vi "add data to plot 1.vi"(8 "error in (no error)":errorcluster, 9 "Input graph":cluster{"Y":dbl[], "Y":dbl[]}[](array[cluster]), 10 "Input Y array":dbl[](array[numeric]), 11 "x":dbl) -> (0 "error in (no error) 2":errorcluster, 3 "Output graph":cluster{dbl[], dbl[]}[](array[cluster]))   [LabVIEW 2024]
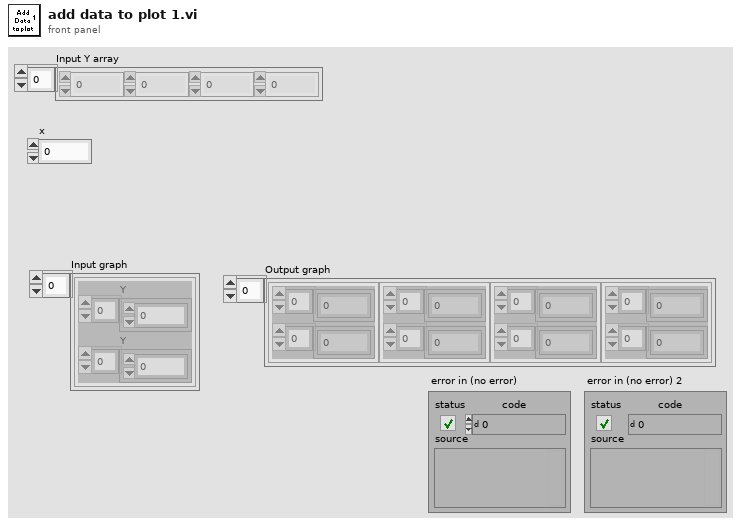
[diagram p1: front panel]
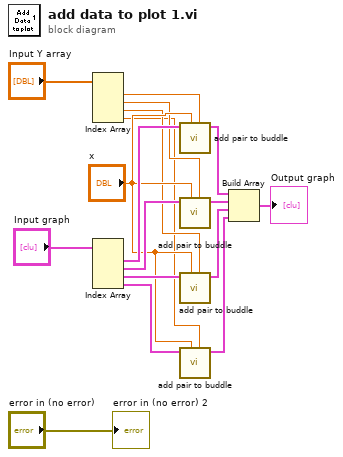
[diagram p0: block diagram]
diagram:
  n1 = Index Array(array="Input Y array") -> (element #1=w6:dbl, element #2=w4:dbl, element #3=w3:dbl, element #4=w2:dbl)  [unwired: 4 in]
  n2 = Index Array(array="Input graph") -> (element #1=w9:cluster{"Y":dbl[], "Y":dbl[]}, element #2=w10:cluster{"Y":dbl[], "Y":dbl[]}, element #3=w11:cluster{"Y":dbl[], "Y":dbl[]}, element #4=w12:cluster{"Y":dbl[], "Y":dbl[]})  [unwired: 4 in]
  n3 = call "add pair to buddle.vi"("y"=w6, "x"="x", "Input"=w9) -> ("output"=w13:cluster{dbl[], dbl[]})  [unwired: 8 in]
  n4 = call "add pair to buddle.vi"("y"=w4, "x"="x", "Input"=w10) -> ("output"=w14:cluster{dbl[], dbl[]})  [unwired: 8 in]
  n5 = call "add pair to buddle.vi"("y"=w3, "x"="x", "Input"=w11) -> ("output"=w15:cluster{dbl[], dbl[]})  [unwired: 8 in]
  n6 = call "add pair to buddle.vi"("y"=w2, "x"="x", "Input"=w12) -> ("output"=w16:cluster{dbl[], dbl[]})  [unwired: 8 in]
  n7 = Build Array(w13, w14, w15, w16) -> (→"Output graph":cluster{dbl[], dbl[]}[])
  "error in (no error) 2" <- "error in (no error)"
